vi "Copy_Sheet_In_Excel 2010.vi"(8 "error in (no error)":errorcluster, 9 "New Sheet Name":string="Sheet4", 10 "Master Sheet Name":string="Sheet1", 11 "Excel Path":path=path "C:/Temp/Test.xlsx") -> (0 "error out":errorcluster)   [LabVIEW 2015]
panel:
  in  "Excel._Worksheet":refnum<k7>
  in  "Excel._Application":refnum<k7>
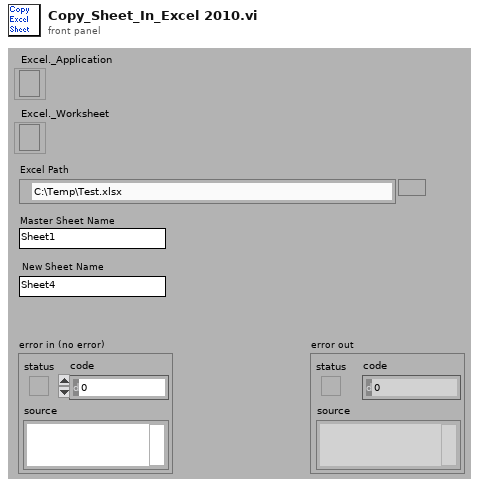
[diagram p1: front panel]
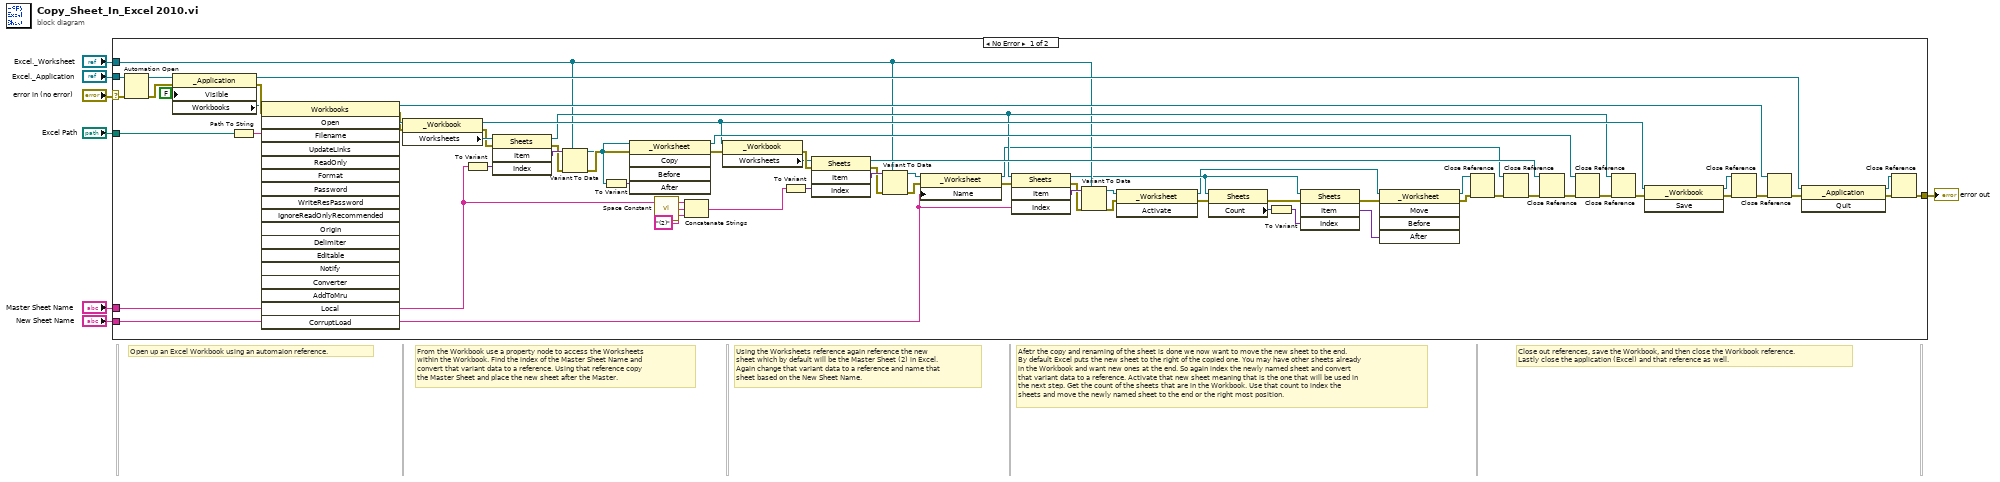
[diagram p0: block diagram]
diagram:
  # "Close out references, save the Workbook, and then close the Workbook reference.\nLastly close the application (Excel) and that reference as well."
  # "Afetr the copy and renaming of the sheet is done we now want to move the new sheet to the end.\nBy default Excel puts the new sheet to the right of the copied one. You may have other sheets already\nin the Workbook and want new ones at the end. So again index the newly named sheet and convert\nthat variant data to a reference. Activate that new sheet meaning that is the one that will be used in\nthe next step. Get the count of the sheets that are in the Workbook. Use that count to index the\nsheets and move the newly named sheet to the end or the right most position."
  # "Using the Worksheets reference again reference the new\nsheet which by default will be the Master Sheet (2) in Excel.\nAgain change that variant data to a reference and name that\nsheet based on the New Sheet Name."
  # "From the Workbook use a property node to access the Worksheets \nwithin the Workbook. Find the index of the Master Sheet Name and \nconvert that variant data to a reference. Using that reference copy\nthe Master Sheet and place the new sheet after the Master."
  # "Open up an Excel Workbook using an automaion reference."
  n1 = case shown="No Error" "error in (no error)" {
    selector: "error in (no error)" -> [w57 w75]
    tunnel: "Excel._Worksheet" -> [w28 _]
    tunnel: [w68 w75] -> w6
    tunnel: "Excel._Application" -> [w64 _]
    tunnel: "Excel Path" -> [w62 _]
    tunnel: "New Sheet Name" -> [w31 _]
    tunnel: "Master Sheet Name" -> [w12 _]
    frame No Error {
      n2 = Automation Open(error in (no error)=w57, Automation Refnum=w64) -> (Automation Refnum=w65:refnum<k7>, error out=w74:errorcluster)  [unwired: 2 out]
      n3 = property class="_Application"(reference=w65, error in=w74, "Visible"=FALSE) -> (reference out=w49:refnum<k7>, error out=w55:errorcluster, "Workbooks"=w54:refnum<k7>)
      n4 = Path To String(path=w62) -> (string=w61:string)
      n5 = invoke class="Workbooks" method="Open"(reference=w54, error in=w55, "Filename"=w61) -> (reference out=w60:refnum<k7>, error out=w58:errorcluster, "Open"=w59:refnum<k7>)  [unwired: 15 in, 15 out]
      n6 = property class="_Workbook"(reference=w59, error in=w58) -> (reference out=w34:refnum<k7>, error out=w52:errorcluster, "Worksheets"=w53:refnum<k7>)
      n7 = To Variant(anything=w12) -> (Variant=w13:variant)
      n8 = invoke class="Sheets" method="Item"(reference=w53, error in=w52, "Index"=w13) -> (reference out=w32:refnum<k7>, error out=w50:errorcluster, "Item"=w51:variant)  [unwired: 1 in, 1 out]
      n9 = Variant To Data(error in=w50, type=w28, Variant=w51) -> (data=w43:refnum<k7>, error out=w48:errorcluster)
      n10 = To Variant(anything=w43) -> (Variant=w47:variant)
      n11 = invoke class="_Worksheet" method="Copy"(reference=w43, error in=w48, "After"=w47) -> (reference out=w36:refnum<k7>, error out=w46:errorcluster)  [unwired: 2 in, 3 out]
      n12 = call <vilib>:"Space Constant.vi"() -> ("String"=w11:string)
      n13 = Concatenate Strings(w12, w11, "(2)") -> (w8:string)
      n14 = property class="_Workbook"(reference=w34, error in=w46) -> (error out=w45:errorcluster, "Worksheets"=w44:refnum<k7>)  [unwired: 1 out]
      n15 = To Variant(anything=w8) -> (Variant=w9:variant)
      n16 = invoke class="Sheets" method="Item"(reference=w44, error in=w45, "Index"=w9) -> (reference out=w37:refnum<k7>, error out=w41:errorcluster, "Item"=w42:variant)  [unwired: 1 in, 1 out]
      n17 = Variant To Data(error in=w41, type=w28, Variant=w42) -> (data=w40:refnum<k7>, error out=w39:errorcluster)
      n18 = property class="_Worksheet"(reference=w40, error in=w39, "Name"=w31) -> (reference out=w17:refnum<k7>, error out=w33:errorcluster)
      n19 = invoke class="Sheets" method="Item"(reference=w32, error in=w33, "Index"=w31) -> (reference out=w24:refnum<k7>, error out=w29:errorcluster, "Item"=w30:variant)  [unwired: 1 in, 1 out]
      n20 = Variant To Data(error in=w29, type=w28, Variant=w30) -> (data=w27:refnum<k7>, error out=w26:errorcluster)
      n21 = invoke class="_Worksheet" method="Activate"(reference=w27, error in=w26) -> (reference out=w19:refnum<k7>, error out=w25:errorcluster)  [unwired: 1 in, 1 out]
      n22 = property class="Sheets"(reference=w24, error in=w25) -> (error out=w23:errorcluster, "Count"=w21:i32)  [unwired: 1 out]
      n23 = To Variant(anything=w21) -> (Variant=w22:variant)
      n24 = invoke class="Sheets" method="Item"(reference=w24, error in=w23, "Index"=w22) -> (error out=w20:errorcluster, "Item"=w18:variant)  [unwired: 1 in, 2 out]
      n25 = invoke class="_Worksheet" method="Move"(reference=w19, error in=w20, "After"=w18) -> (reference out=w14:refnum<k7>, error out=w15:errorcluster)  [unwired: 2 in, 3 out]
      n26 = Close Reference(reference=w14, error in (no error)=w15) -> (error out=w16:errorcluster)
      n27 = Close Reference(reference=w17, error in (no error)=w16) -> (error out=w38:errorcluster)
      n28 = Close Reference(reference=w37, error in (no error)=w38) -> (error out=w35:errorcluster)
      n29 = Close Reference(reference=w36, error in (no error)=w35) -> (error out=w56:errorcluster)
      n30 = Close Reference(reference=w32, error in (no error)=w56) -> (error out=w63:errorcluster)
      n31 = invoke class="_Workbook" method="Save"(reference=w34, error in=w63) -> (reference out=w71:refnum<k7>, error out=w72:errorcluster)  [unwired: 1 in, 1 out]
      n32 = Close Reference(reference=w71, error in (no error)=w72) -> (error out=w70:errorcluster)
      n33 = Close Reference(reference=w60, error in (no error)=w70) -> (error out=w67:errorcluster)
      n34 = invoke class="_Application" method="Quit"(reference=w49, error in=w67) -> (reference out=w66:refnum<k7>, error out=w69:errorcluster)  [unwired: 1 in, 1 out]
      n35 = Close Reference(reference=w66, error in (no error)=w69) -> (error out=w68:errorcluster)
    }
    frame Error {
    }
  }
  "error out" <- w6
